vi "PID.vi"(11 "PID gains":T1={"proportional gain (Kc)"=0.021, "integral time (Ti, min)"=0.0, "derivative time (Td, min)"=0.0} {"derivative time (Td, min)" format="%.3f"; "integral time (Ti, min)" format="%.3f"; "proportional gain (Kc)" format="%.3f"}) -> (3 "output":dbl)   [LabVIEW 2014]
uses:
  <vilib>/addons/control/pid/pid.llb/PID (DBL).vi
  _2015 Season/Mecanum Prototype v5/Mecanum Prototype v1/Robot Global Data.vi
  <vilib>/addons/control/pid/NI_PID_pid.lvlib
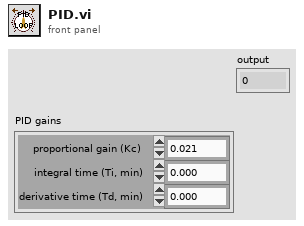
[diagram p1: front panel]
types:
  T1 = cluster{"proportional gain (Kc)":dbl, "integral time (Ti, min)":dbl, "derivative time (Td, min)":dbl}
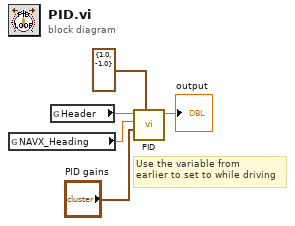
[diagram p0: block diagram]
diagram:
  # "Use the variable from\nearlier to set to while driving"
  n1 = global read "Robot Global Data.vi" "NAVX_Heading"() -> (w5:dbl)
  n2 = global read "Robot Global Data.vi" "Header"() -> (w1:dbl)
  n3 = call-poly <vilib>:"PID.vi"("output range"=cluster{"output high":dbl, "output low":dbl} {"output high"=1.0, "output low"=-1.0}, "PID gains"="PID gains", "process variable"=w5, "setpoint"=w1) -> ("output"=→"output":dbl)  [unwired: 6 in, 1 out]
